vi "IC measurment N6972A - Rohan version - 24.06 WHILELOOP.vi"() -> ()   [LabVIEW 2022 SP3]
doc: "This example demonstrates how to configure a list in current priority mode."
uses:
  <vilib>/Analysis/baseanly.llb/Mean (DBL).vi
  <instrlib>/Agilent 34420/Public/Data/Read (Multiple Points).vi
  <instrlib>/Agilent N6900 N7900 Series/Agilent N6900 N7900 Series.lvlib
  <instrlib>/Agilent 34420/Agilent 34420.lvlib
  <vilib>/Analysis/NI_AALBase.lvlib
  <vilib>/Utility/TDMS File Viewer/NI_TDMS File Viewer.lvlib
panel:
  out "Boolean":bool
  out "String":string="WARNING: FILE PATH EXISTS"
  in  "Path":path=path "C:/Users/kumarr3/OneDrive - Victoria University of Wellington - STAFF/Documents/DataFiles/NoLoad" caption="Load File Path or Directory"
  in  "Conduct Experiment\n\n\nLoad Experiment":bool
  in  "relative path (file or folder)":path=path "Test.tdms"
  in  "base path":path=path "C:/Users/kumarr3/OneDrive - Victoria University of Wellington - STAFF/Documents/DataFiles"
  in  "Tab Control":T1(tab)
  in  "N6972A VISA resource name":refnum<visa-resource-name>="USB0::0x0957::0x3407::MY63000447::INSTR"
  in  "Current Priority Voltage Limit":dbl=1.0
  in  "34420A VISA resource name":refnum<visa-resource-name>="COM3"
  in  "Resolution (1E-9)":dbl=1e-09
  in  "Manual Range (0.001)":dbl=0.001
  in  "Auto Range (T: Enable)":bool=TRUE
  in  "Serial Configuration":T2={"Baud Rate"=9600, "Parity"=0, "Data Bits"=8} {"Data Bits" items=["7"=7, "8"=8]; "Parity" items=["None", "Odd", "Even", "Mark", "Space"]; "Baud Rate" items=["300"=300, "600"=600, "1200"=1200, "2400"=2400, "4800"=4800, "9600"=9600]}
  in  "Function (0: DC Volts)":u16(ring) items=["DC Volts", "DC Voltage Ratio", "DC Voltage Difference", "2 Wire Resistance", "4 Wire Resistance", "Temperature"]
  in  "Channel (1: Channel 1)":u16(ring)=1 items=["Channel 1"=1, "Channel 2"=2]
  in  "Filter On/Off":string(combo)="OFF"
  in  "Voltmeter Offset Sample Count":i32=10
  in  "Integration Time (4: 10 NPLCs)":u16(ring)=4 items=["0.02 NPLC", "0.2 NPLC", "1 NPLC", "2 NPLCs", "10 NPLCs", "20 NPLCs", "100 NPLCs", "200 NPLCs"]
  out "CURRENT RUN":string
  out "Waveform Chart":dbl(graph)
  in  "Measure Temperature?":bool
  out "Temperature Chart":dbl[](graph)=[25.735546538805686]
  out "?":string
  out "Progress Bar":dbl(slide) scale=0.0..1000.0
  in  "Minutes  / Seconds":bool
  in  "Hours / Minutes":bool
  in  "RUN MULTIPLE MEASUREMENTS":bool
  in  "Measurement Interval":dbl
  in  "Total Measurement Time":dbl
  out "XY Graph":cluster{dbl[], dbl[]}(graph)
  out "RMS Current":dbl
  out "uV/cm":dbl
  out "Voltmeter offset (µV)":dbl format="%e"
  out "Current array":dbl[](array[numeric])
  out "Voltage  array":dbl[](array[numeric])
  out "?":bool
  in  "Volt. Tap threshold (uV/cm)":dbl=0.25 format="%.2f"
  in  "Current increment above µV threshold [A]":dbl=0.1 format="%.2f"
  out "?":bool
  in  "Current increment 2 [A]":dbl=0.2 format="%.2f"
  in  "Current limit 1 [A]":dbl=38.0 format="%.2f"
  in  "Initial Current increment  [A]":dbl=5.0 format="%.2f"
  out "Max volt. reached":bool
  out "Max. current reached":bool
  in  "Max. Volt. Tap Voltage (uV/cm)":dbl=10.0
  in  "Maximum current (A)":dbl=48.0
  in  "Volt. Tap Distance (cm)":dbl=1.6
  in  "stop":bool
  out "Calibrating Offset?":bool
  out "Offset V vals":dbl[](array[numeric])
  out "Terminated Temp Msre":bool=TRUE
  in  "Temperature Reading Iterval(s)":u32=1
  in  "Ramp interval (s)":u32
  out "Start Time":timestamp
  out "Experiment Elapsed Time":string
  out "Experiment Remaining Time":string
  out "Waiting time elapsed":string
  in  "Number of Repeats":i32=1
  out "n Values":cluster{timestamp[], dbl[]}(graph)
  out "Ic Values":cluster{timestamp[], dbl[]}(graph)
  out "Fitting Status":string
  out "median Ic":dbl format="%0.2f"
  out "Current Run":cluster{dbl[], dbl[]}(graph) caption="XY Graph"
  out "Historial Results":cluster{dbl[], dbl[]}[](graph) caption="XY Graph"
  out "Ic Array":dbl[](array[numeric])
  out "n Array":dbl[](array[numeric])
  out "mean Ic":dbl format="%0.2f"
  out "mean n":dbl format="%0.2f"
  out "median n":dbl format="%0.2f"
  out "XY Graph 2":cluster{timestamp[], dbl[]}(graph)
  out "median n":dbl format="%0.2f"
  out "n Values Graph":cluster{timestamp[], dbl[]}(graph)
  out "Ic Values Graph":cluster{timestamp[], dbl[]}(graph)
  out "n Array":dbl[](array[numeric])
  out "Ic Array":dbl[](array[numeric])
  out "mean n":dbl format="%0.2f"
  out "mean Ic (A)":dbl format="%0.2f"
  out "Historical Data":cluster{"Array":dbl[], "Array":dbl[]}[](graph)
  out "Number of Runs":dbl
  out "Experiment Description":variant
  out "median Ic (A)":dbl format="%0.2f"
  out "current time":timestamp
  # "Ic Test Controls"
  # "Experiment Control"
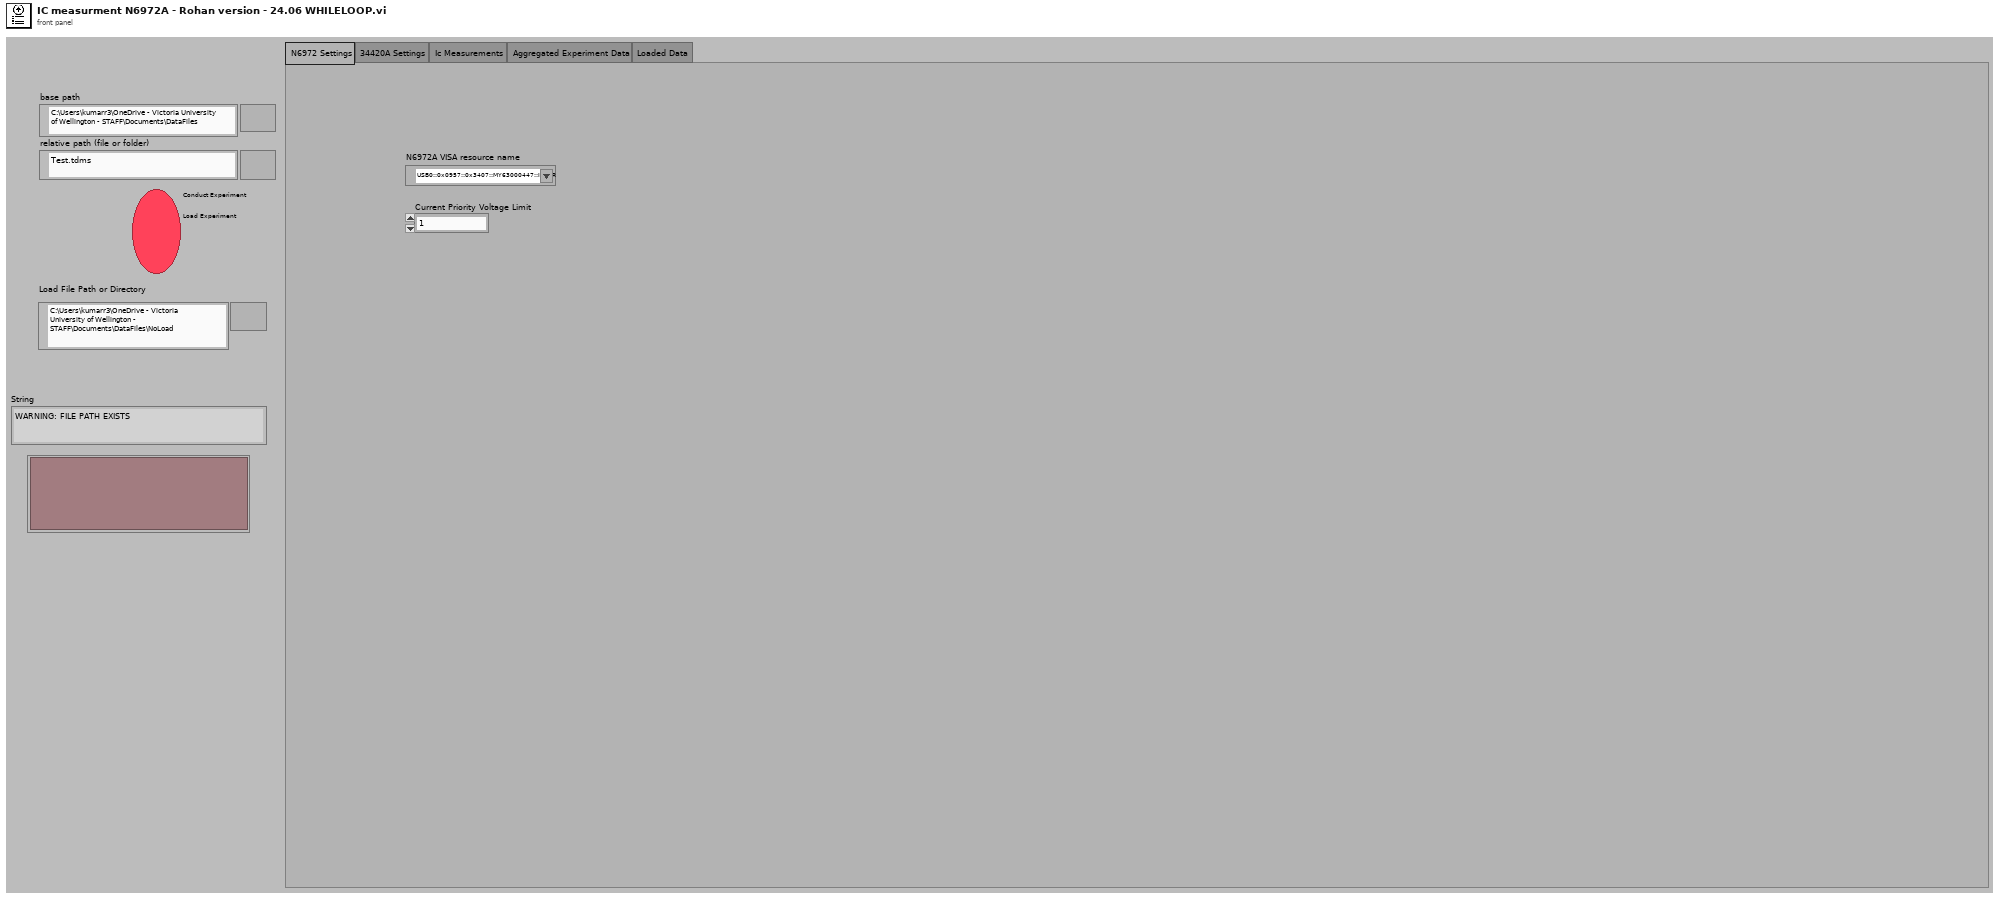
[diagram p1: front panel]
types:
  T1 = enum32{"N6972 Settings", "34420A Settings", "Ic Measurements", "Aggregated Experiment Data", "Loaded Data"}
  T2 = cluster{"Baud Rate":u32, "Parity":u16, "Data Bits":u16}
  T3 = enum16{"open", "open or create", "create or replace", "create", "open (read-only)"}
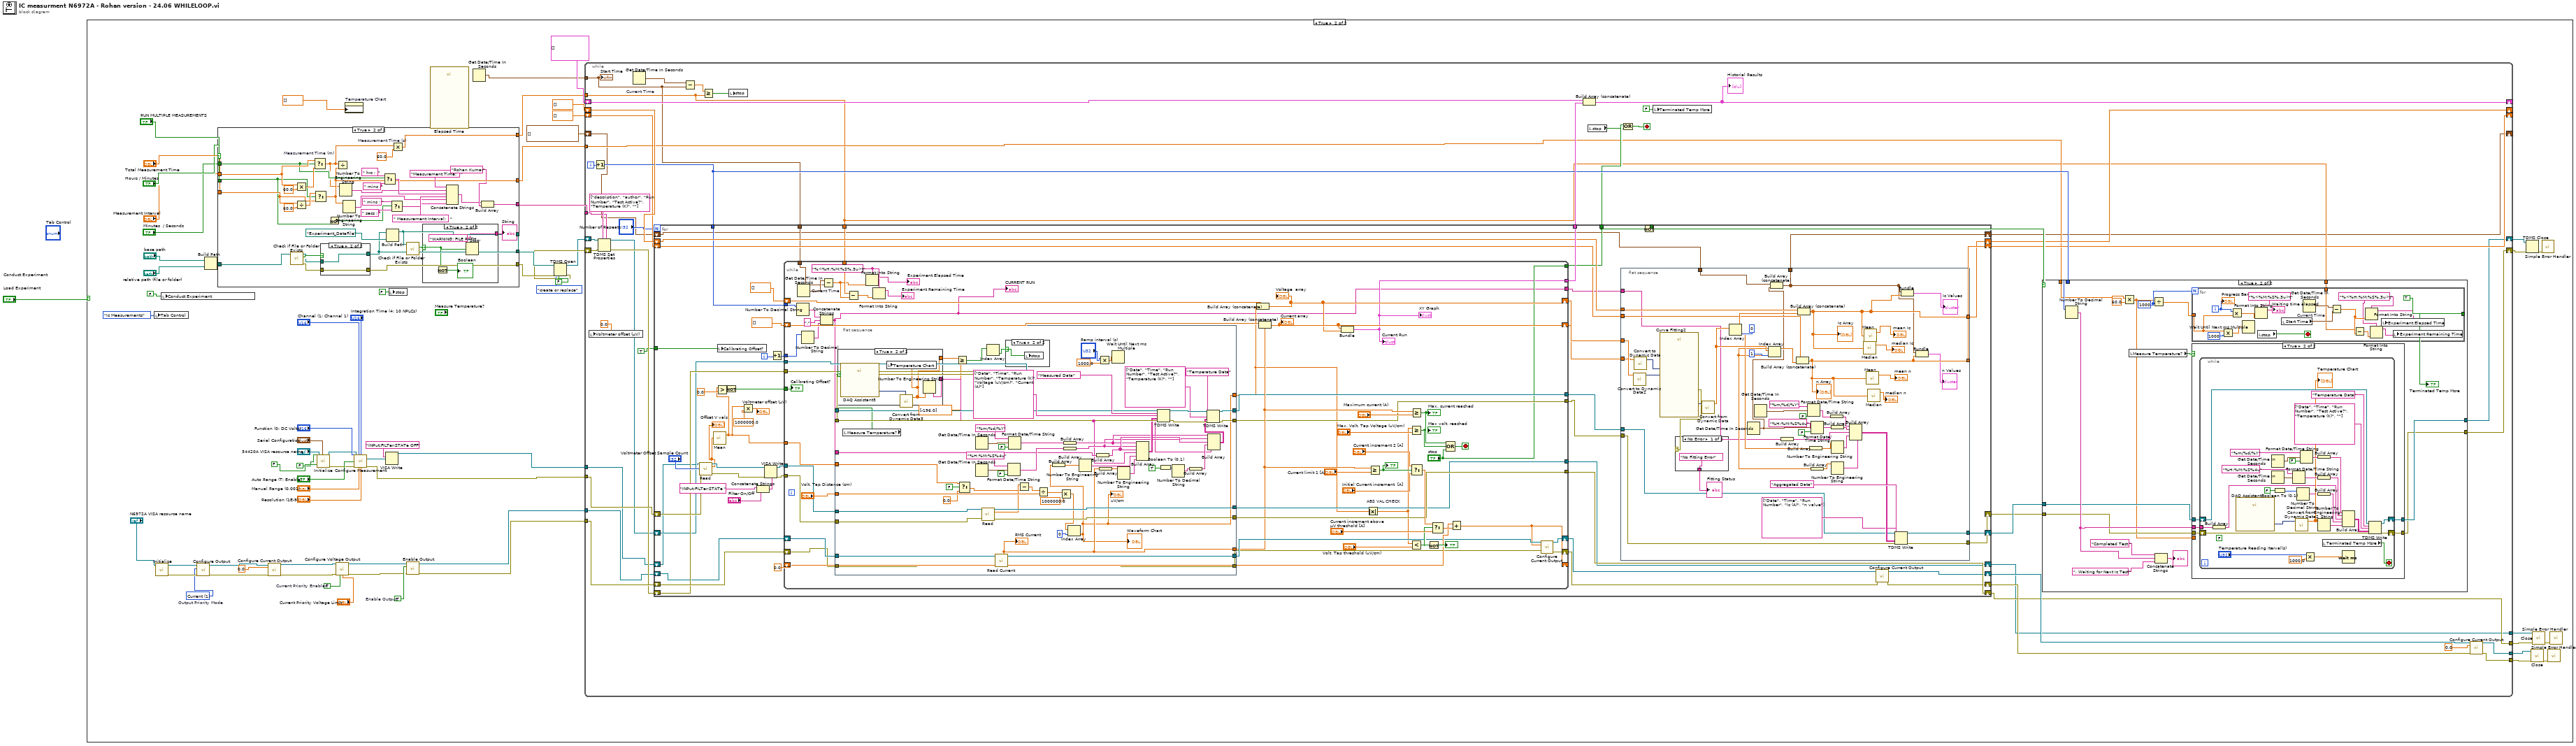
[diagram p0: block diagram]
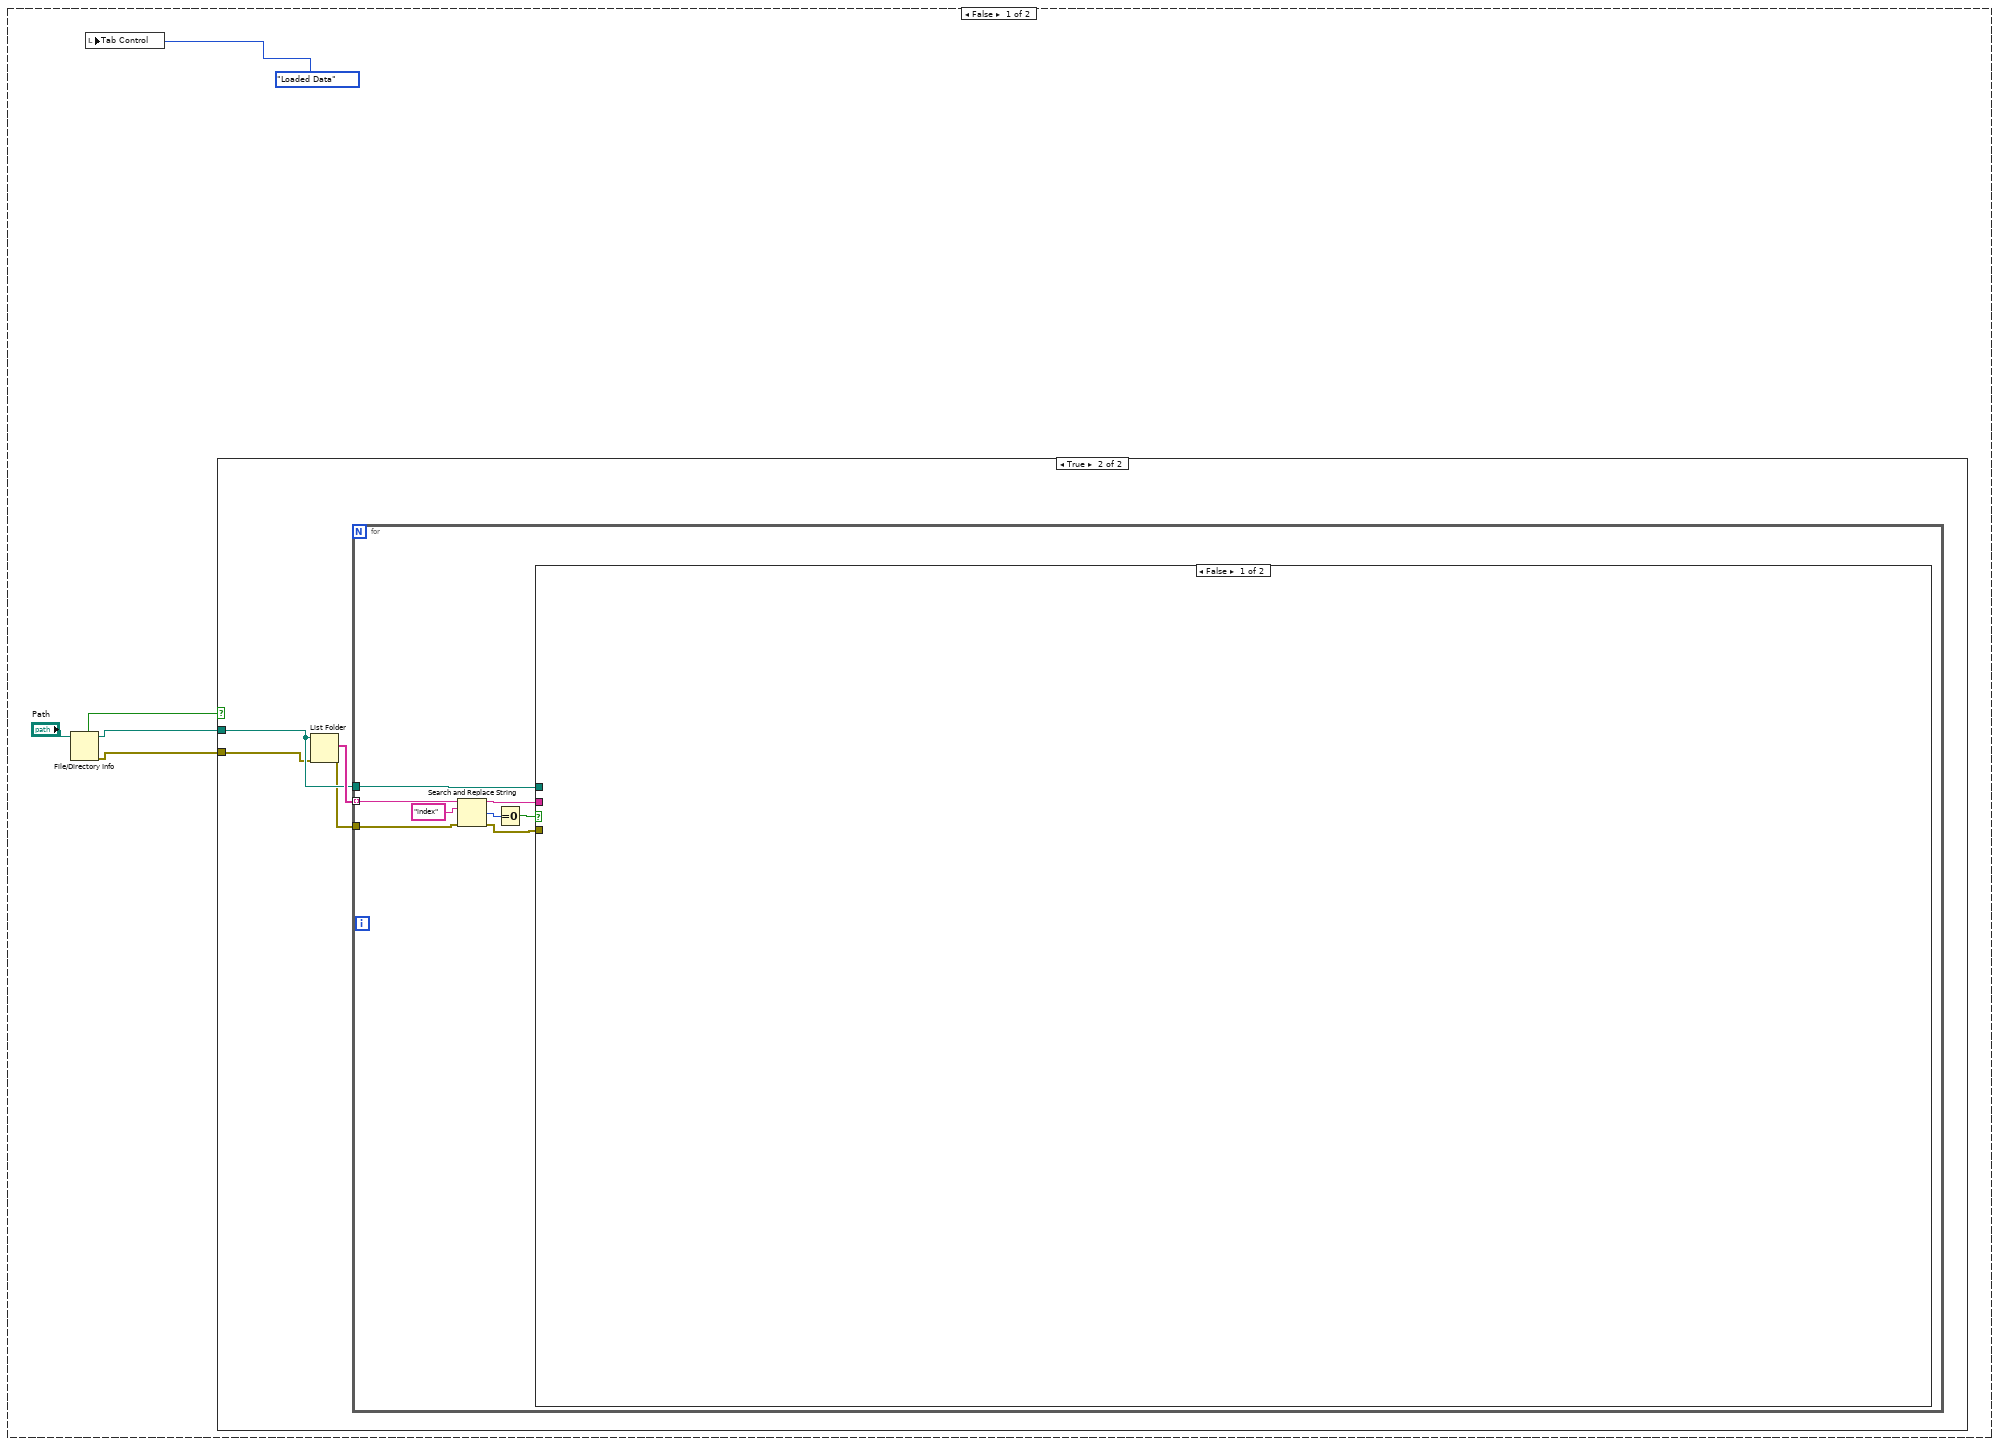
[diagram p2: hidden frame]
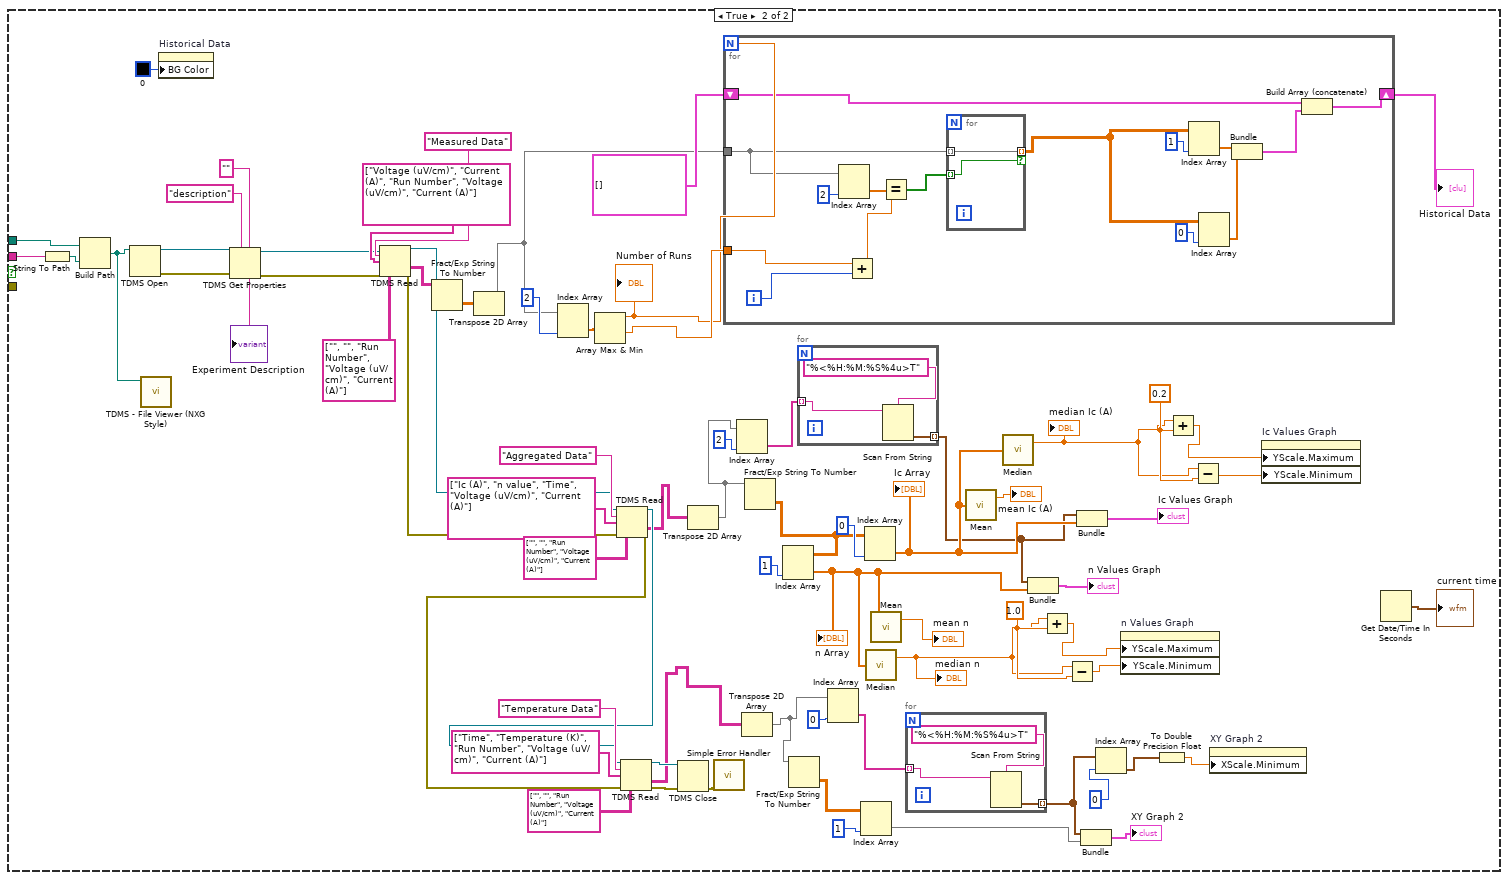
[diagram p4: hidden frame]
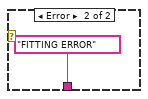
[diagram p5: hidden frame]
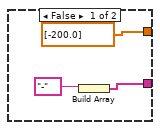
[diagram p7: hidden frame]
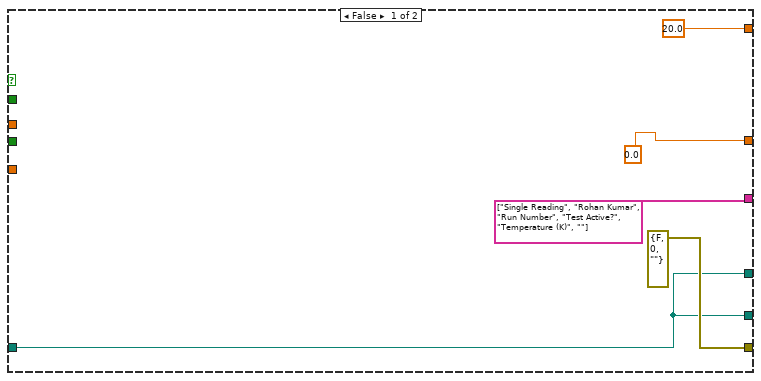
[diagram p10: hidden frame]
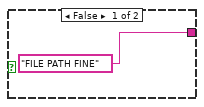
[diagram p11: hidden frame]
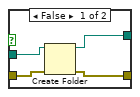
[diagram p12: hidden frame]
diagram:
  n1 = case shown="True" "Conduct Experiment\n\n\nLoad Experiment" {
    frame False {
      n2 = File/Directory Info(path="Path") -> (path out=w5:path, directory=w4:bool, error out=w3:errorcluster)  [unwired: 1 in, 4 out]
      n3 = local write "Tab Control"(T1."Loaded Data" ("Tab Control")) -> ()
      n4 = case shown="True" w4 {
        tunnel: w5 -> [_ w9]
        tunnel: w3 -> [_ w8]
        frame False {
        }
        frame True {
          n5 = List Folder(path=w9, error in=w8) -> (filenames=w10:string[], error out=w7:errorcluster)  [unwired: 2 in, 2 out]
          n6 = for {
            tunnel: w10 -> [w18] mode=indexing
            tunnel: w9 -> [w14]
            tunnel: w7 -> [w12]
            n7 = Search and Replace String(input string=w18, search string="index", error in=w12) -> (result string=w13:string, number of replacements=w16:i32, error out=w11:errorcluster)  [unwired: 5 in, 1 out]
            n8 = Equal To 0?(x=w16) -> (x = 0?=w15:bool)
            n9 = case shown="False" w15 {
              tunnel: w13 -> [_ w90]
              tunnel: w14 -> [_ w89]
              tunnel: w11 -> [_ _]
              frame False {
              }
              frame True {
                w27 = 1.0
                w29 = 0.2
                n10 = String To Path(string=w90) -> (path=w88:path)
                n11 = Build Path(base path=w89, name or relative path=w88) -> (appended path=w19:path)
                n12 = TDMS Open(11:w19) -> (0:w66:errorcluster, 3:w67:refnum<k34>)  [unwired: 6 in]
                n13 = call <vilib>:"TDMS - File Viewer (NXG Style).vi"("file in"=w19) -> ()  [unwired: 9 in, 2 out]
                n14 = property on="Historical Data" class="XYGraph (strict)"("BG Color"=u32 0 ("Plot Area:Colors:BG Color")) -> ()  [unwired: 2 in, 2 out]
                n15 = TDMS Get Properties(5:"", 7:"description", 8:w66, 11:w67) -> (0:w64:errorcluster, 3:w65:refnum<k34>, 4:→"Experiment Description":string)  [unwired: 2 in, 3 out]
                n16 = TDMS Read(0:w65, 5:"Measured Data" ("group name in"), 7:string[] ["Voltage (uV/cm)", "Current (A)", "Run Number", "Voltage (uV/cm)", "Current (A)"] ("channel name(s) in (Untitled)"), 11:w64, 12:string[][] [["", "", "Run Number", "Voltage (uV/cm)", "Current (A)"]] ("channel name(s) in (Untitled)")) -> (4:w54:refnum<k34>, 10:w84:string[][], 15:w53:errorcluster)  [unwired: 3 in, 3 out]
                n17 = Fract/Exp String To Number(string=w84) -> (number=w83:dbl[][])  [unwired: 3 in, 1 out]
                n18 = Transpose 2D Array(2D array=w83) -> (transposed array=w69:dbl[][])
                n19 = Index Array(array=w69, index (col)=2 ("disabled index (col)")) -> (element=w74:dbl[])  [unwired: 1 in]
                n20 = Array Max & Min(array=w74) -> (max value=w72:dbl, min value=w73:dbl)  [unwired: 2 out]
                "Number of Runs" <- w72
                n21 = TDMS Read(0:w54, 5:"Aggregated Data" ("group name in"), 7:string[] ["Ic (A)", "n value", "Time", "Voltage (uV/cm)", "Current (A)"] ("channel name(s) in (Untitled)"), 11:w53, 12:string[][] [["", "", "Run Number", "Voltage (uV/cm)", "Current (A)"]] ("channel name(s) in (Untitled)")) -> (4:w52:refnum<k34>, 10:w34:string[][], 15:w51:errorcluster)  [unwired: 3 in, 3 out]
                n22 = TDMS Read(0:w52, 5:"Temperature Data" ("group name in"), 7:string[] ["Time", "Temperature (K)", "Run Number", "Voltage (uV/cm)", "Current (A)"] ("channel name(s) in (Untitled)"), 11:w51, 12:string[][] [["", "", "Run Number", "Voltage (uV/cm)", "Current (A)"]] ("channel name(s) in (Untitled)")) -> (4:w56:refnum<k34>, 10:w48:string[][], 15:w55:errorcluster)  [unwired: 3 in, 3 out]
                n23 = TDMS Close(8:w55, 11:w56) -> (0:w60:errorcluster)  [unwired: 1 out]
                n24 = Transpose 2D Array(2D array=w34) -> (transposed array=w33:string[][])
                n25 = call <vilib>:"Simple Error Handler.vi"("error in (no error)"=w60) -> ()  [unwired: 2 in, 7 out]
                n26 = for {
                  N: w72 -> [_]
                  tunnel: w69 -> [w105]
                  tunnel: w73 -> [w103]
                  shift-right: [w97] -> w70
                  shift-left: cluster{dbl[], dbl[]}[] [] -> [w99]
                  i -> [w111]
                  n27 = Index Array(array=w105, index (col)=2 ("disabled index (col)")) -> (element=w106:dbl[])  [unwired: 1 in]
                  n28 = Add(x=w103, y=w111) -> (x+y=w104:dbl)
                  n29 = Equal?(x=w106, y=w104) -> (x = y?=w101:bool[])
                  n30 = for {
                    tunnel: w101 -> [w112] mode=indexing
                    tunnel: w105 -> [w113] mode=indexing
                    tunnel: [w113] -> w102 mode=indexing if=w112
                  }
                  n31 = Index Array(array=w102, index (col)=1 ("disabled index (col)")) -> (element=w108:dbl[])  [unwired: 1 in]
                  n32 = Index Array(array=w102, index (col)=0 ("disabled index (col)")) -> (element=w107:dbl[])  [unwired: 1 in]
                  n33 = Bundle(w108, w107) -> (w98:cluster{dbl[], dbl[]})  [unwired: 1 in]
                  n34 = Build Array (concatenate)(w99, w98) -> (w97:cluster{dbl[], dbl[]}[])
                }
                "Historical Data" <- w70
                n35 = Index Array(array=w33, index (col)=2 ("disabled index (col)")) -> (element=w40:string[])  [unwired: 1 in]
                n36 = Transpose 2D Array(2D array=w48) -> (transposed array=w45:string[][])
                n37 = Fract/Exp String To Number(string=w33) -> (number=w32:dbl[][])  [unwired: 3 in, 1 out]
                n38 = Index Array(array=w32, index (col)=1 ("disabled index (col)")) -> (element=w39:dbl[])  [unwired: 1 in]
                "n Array" <- w39
                n39 = Fract/Exp String To Number(string=w45) -> (number=w47:dbl[][])  [unwired: 3 in, 1 out]
                n40 = for {
                  tunnel: w40 -> [w93] mode=indexing
                  tunnel: [w91] -> w36 mode=indexing
                  n41 = Scan From String(format string="%<%H:%M:%S%4u>T" ("time format string (%c)"), input string=w93) -> (output 1=w91:timestamp)  [unwired: 3 in, 3 out]
                }
                n42 = Index Array(array=w45, index (col)=0 ("disabled index (col)")) -> (element=w44:string[])  [unwired: 1 in]
                n43 = Index Array(array=w47, index (col)=1 ("disabled index (col)")) -> (element=w43:dbl[])  [unwired: 1 in]
                n44 = Index Array(array=w32, index (col)=0 ("disabled index (col)")) -> (element=w37:dbl[])  [unwired: 1 in]
                "Ic Array" <- w37
                n45 = call <vilib>:"Median.vi"("X"=w39) -> ("median"=w24:dbl)  [unwired: 1 out]
                "median n" <- w24
                n46 = call-poly <vilib>:"Mean.vi"("X"=w39) -> ("mean"=→"mean n":dbl)  [unwired: 1 out]
                n47 = for {
                  tunnel: w44 -> [w96] mode=indexing
                  tunnel: [w94] -> w23 mode=indexing
                  n48 = Scan From String(format string="%<%H:%M:%S%4u>T" ("time format string (%c)"), input string=w96) -> (output 1=w94:timestamp)  [unwired: 3 in, 3 out]
                }
                n49 = call-poly <vilib>:"Mean.vi"("X"=w37) -> ("mean"=→"mean Ic (A)":dbl)  [unwired: 1 out]
                n50 = call <vilib>:"Median.vi"("X"=w37) -> ("median"=w28:dbl)  [unwired: 1 out]
                "median Ic (A)" <- w28
                n51 = Bundle(w36, w39) -> (→"n Values Graph":cluster{timestamp[], dbl[]})  [unwired: 1 in]
                n52 = Add(x=w24, y=w27) -> (x+y=w26:dbl)
                n53 = Subtract(x=w24, y=w27) -> (x-y=w25:dbl)
                n54 = Bundle(w36, w37) -> (→"Ic Values Graph":cluster{timestamp[], dbl[]})  [unwired: 1 in]
                n55 = Bundle(w23, w43) -> (→"XY Graph 2":cluster{timestamp[], dbl[]})  [unwired: 1 in]
                n56 = Index Array(array=w23, index=0 ("disabled index (col)")) -> (element=w21:timestamp)
                n57 = property on="n Values Graph" class="XYGraph (strict)"("YScale.Maximum"=w26, "YScale.Minimum"=w25) -> ()  [unwired: 2 in, 2 out]
                n58 = To Double Precision Float(number=w21) -> (double precision float=w20:dbl)
                n59 = Add(x=w28, y=w29) -> (x+y=w30:dbl)
                n60 = Subtract(x=w28, y=w29) -> (x-y=w31:dbl)
                n61 = property on="XY Graph 2" class="XYGraph (strict)"("XScale.Minimum"=w20) -> ()  [unwired: 2 in, 2 out]
                n62 = property on="Ic Values Graph" class="XYGraph (strict)"("YScale.Maximum"=w30, "YScale.Minimum"=w31) -> ()  [unwired: 2 in, 2 out]
                n63 = Get Date/Time In Seconds() -> (seconds since 1Jan1904=→"current time":timestamp)
              }
            }
          }
        }
      }
    }
    frame True {
      w174 = TRUE  # Enable Output
      w171 = TRUE  # Current Priority Enabled
      w178 = u16 1 items=["Voltage", "Current"]  # Output Priority Mode
      n64 = local write "Tab Control"(T1."Ic Measurements" ("Tab Control")) -> ()
      n65 = call <instrlib>:"Initialize.vi"("VISA resource name"="N6972A VISA resource name") -> ("error out"=w179:errorcluster, "VISA resource name out"=w180:refnum<visa-resource-name>)  [unwired: 9 in]
      n66 = local write "Conduct Experiment\n\n\nLoad Experiment"(FALSE) -> ()
      n67 = call <instrlib>:"Configure Output.vi"("error in (no error)"=w179, "Output Priority Mode (0: Voltage)"=w178, "VISA resource name"=w180) -> ("error out"=w176:errorcluster, "VISA resource name out"=w177:refnum<visa-resource-name>)  [unwired: 7 in]
      n68 = Build Path(base path="base path", name or relative path="relative path (file or folder)") -> (appended path=w133:path)
      n69 = case shown="True" "RUN MULTIPLE MEASUREMENTS" {
        tunnel: "Total Measurement Time" -> [_ w558]
        tunnel: "Measurement Interval" -> [_ w555]
        tunnel: [0.0 ("Measurement Interval (Minutes)") w544] -> w132
        tunnel: w133 -> [w528 w564]
        tunnel: [w528 w538] -> w127
        tunnel: [errorcluster {"status"=FALSE, "code"=0, "source"=""} ("error out") w561] -> w129
        tunnel: "Hours / Minutes" -> [_ w545]
        tunnel: "Minutes  / Seconds" -> [_ w535]
        tunnel: [w528 w554] -> _
        tunnel: [string[] ["Single Reading", "Rohan Kumar", "Run Number", "Test Active?", "Temperature (K)", ""] ("channel name(s) in (Untitled)") w539] -> w120
        tunnel: [20.0 ("Measurement Interval (Minutes)") w532] -> w115
        frame False {
        }
        frame True {
          n70 = call <vilib>:"Check if File or Folder Exists.vi"("path"=w564) -> ("error out"=w562:errorcluster, "file or folder exists?"=w563:bool, "dup path"=w560:path)  [unwired: 8 in]
          n71 = Multiply(x=w558, y=60.0) -> (x*y=w557:dbl)
          n72 = Divide(x=w555, y=60.0) -> (x/y=w556:dbl)
          n73 = Select "Measurement Time (m)"(t=w558, s=w545, f=w557) -> (s? t:f=w531:dbl)
          n74 = Select(t=w556, s=w535, f=w555) -> (s? t:f=w544:dbl)
          n75 = case shown="True" w563 {
            tunnel: w562 -> [w574 w575]
            tunnel: [w573 w575] -> w561
            tunnel: [w572 w576] -> w554
            tunnel: w560 -> [w571 w576]
            frame False {
              n76 = Create Folder(path (use dialog)=w571, error in=w574) -> (created path=w572:path, error out=w573:errorcluster)  [unwired: 1 in, 1 out]
            }
            frame True {
            }
          }
          n77 = Not(x=w535) -> (.not. x?=w534:bool)
          n78 = Divide(x=w531, y=w544) -> ()  [unwired: 1 out]
          n79 = Number To Engineering String(4:w531) -> (0:w542:string)  [unwired: 3 in]
          n80 = Number To Engineering String(4:w544) -> (0:w543:string)  [unwired: 3 in]
          n81 = Select(t=" hrs ;  ", s=w545, f=" mins ;") -> (s? t:f=w548:string)
          n82 = Build Path(base path=w554, name or relative path=path "Experiment_DataFile") -> (appended path=w538:path)
          n83 = Select(t=" mins ; ", s=w534, f=" secs ; ") -> (s? t:f=w546:string)
          n84 = Multiply "Measurement Time (s)"(x=w531, y=60.0) -> (x*y=w532:dbl)
          n85 = call <vilib>:"Check if File or Folder Exists.vi"("path"=w538) -> ("file or folder exists?"=w537:bool)  [unwired: 8 in, 2 out]
          n86 = case shown="True" w537 {
            selector: w537 -> [_ w569]
            tunnel: ["FILE PATH FINE" "WARNING: FILE PATH EXISTS"] -> w536
            frame False {
            }
            frame True {
              n87 = Not(x=w569) -> (.not. x?=→"Boolean":bool)
              n88 = Stop(stop? (T)=w569) -> ()
            }
          }
          "String" <- w536
          n89 = Concatenate Strings("Measurement Time:   ", w542, w548, " Measurement Interval:   ", w543, w546) -> (w540:string)
          n90 = Build Array(w540, "Rohan Kumar") -> (w539:string[])
        }
      }
      n91 = call <instrlib>:"Configure Current Output.vi"("VISA resource name"=w177, "Current Immediate Amplitude (0 A)"=0.0, "error in (no error)"=w176) -> ("VISA resource name out"=w172:refnum<visa-resource-name>, "error out"=w173:errorcluster)  [unwired: 11 in]
      n92 = call <instrlib>:"Initialize.vi"("Serial Configuration"="Serial Configuration", "Reset (True)"=FALSE, "ID Query (True)"=FALSE, "VISA resource name"="34420A VISA resource name") -> ("error out"=w162:errorcluster, "VISA resource name out"=w161:refnum<visa-resource-name>)  [unwired: 6 in]
      n93 = call <instrlib>:"Configure Voltage Output.vi"("VISA resource name"=w172, "error in (no error)"=w173, "Enable Current Priority (False)"=w171, "Current Priority Voltage Limit (25V)"="Current Priority Voltage Limit") -> ("VISA resource name out"=w169:refnum<visa-resource-name>, "error out"=w168:errorcluster)  [unwired: 10 in]
      n94 = property on="Temperature Chart" class="WFChart (strict)"("History Data"=dbl[] []) -> ()  [unwired: 2 in, 2 out]
      n95 = call <instrlib>:"Configure Measurement.vi"("VISA resource name"=w161, "Channel (1: Channel 1)"="Channel (1: Channel 1)", "Integration Time (4: 10 NPLCs)"="Integration Time (4: 10 NPLCs)", "Function (0: DC Volts)"="Function (0: DC Volts)", "Auto Range (T:Enable)"="Auto Range (T: Enable)", "error in (no error)"=w162, "Manual Range (0.001)"="Manual Range (0.001)", "Resolution (1E-9)"="Resolution (1E-9)") -> ("VISA resource name out"=w156:refnum<visa-resource-name>, "error out"=w149:errorcluster)  [unwired: 6 in]
      n96 = VISA Write(VISA resource name=w156, write buffer="INPut:FILTer:STATe OFF") -> (VISA resource name out=w150:refnum<visa-resource-name>)  [unwired: 1 in, 2 out]
      n97 = local write "stop"(FALSE ("stop")) -> ()
      n98 = call <instrlib>:"Enable Output.vi"("error in (no error)"=w168, "Enable Output (F: Disable)"=w174, "VISA resource name"=w169) -> ("error out"=w153:errorcluster, "VISA resource name out"=w154:refnum<visa-resource-name>)  [unwired: 7 in]
      n99 = call "Elapsed Time"() -> ()  [unwired: 12 in, 8 out]
      n100 = Get Date/Time In Seconds() -> (seconds since 1Jan1904=w116:timestamp)
      n101 = TDMS Open(6:FALSE ("disable buffering (T)"), 8:w129, 10:T3."create or replace" ("operation"), 11:w127) -> (0:w126:errorcluster, 3:w125:refnum<k34>)  [unwired: 3 in]
      n102 = while {
        tunnel: w154 -> [w184]
        tunnel: w153 -> [w223]
        tunnel: w132 -> [w192]
        tunnel: w150 -> [w185]
        tunnel: w149 -> [w221]
        tunnel: [w220] -> w147
        tunnel: [w219] -> w146
        tunnel: [w218] -> w144
        tunnel: [w213] -> w143
        shift-right: [w197] -> _
        shift-left: cluster{dbl[], dbl[]}[] [] -> [w215]
        shift-right: [w200] -> _
        shift-left: dbl[] [] -> [w214]
        shift-right: [w201] -> _
        shift-left: dbl[] [] -> [w198]
        shift-right: [w195] -> w124
        shift-left: w125 -> [w207]
        shift-right: [w196] -> w131
        shift-left: w126 -> [w206]
        tunnel: w120 -> [w202]
        tunnel: w116 -> [w188]
        tunnel: w115 -> [w187]
        shift-right: [w182] -> _
        shift-left: timestamp[] [] -> [w183]
        i -> [w217]
        stop <- w209 stop-if-true
        n103 = local write "Voltmeter offset (µV)"(0.0 ("Voltmeter offset (v)")) -> ()
        n104 = Increment(x=w217) -> (x+1=w211:i32)
        n105 = TDMS Set Properties(5:w202, 7:string[] ["description", "author", "Run Number", "Test Active?", "Temperature (K)", ""] ("channel name(s) in (Untitled)"), 8:w206, 11:w207) -> (0:w205:errorcluster, 3:w204:refnum<k34>)  [unwired: 2 in, 2 out]
        n106 = Get Date/Time In Seconds "Current Time"() -> (seconds since 1Jan1904=w191:timestamp)
        n107 = for {
          N: "Number of Repeats" -> [_]
          tunnel: [w263] -> w216
          tunnel: [w258] -> w212
          tunnel: w211 -> [w257]
          tunnel: [w255] -> w210
          tunnel: w188 -> [w241]
          tunnel: w187 -> [w240]
          shift-right: [w236] -> w225
          shift-left: w223 -> [w275]
          shift-right: [w242] -> w193
          shift-left: w221 -> [w267]
          shift-right: [w264] -> w218
          shift-left: w205 -> [w254]
          shift-right: [w243] -> w194
          shift-left: w204 -> [w253]
          shift-right: [w252] -> w201
          shift-left: w198 -> [w246]
          shift-right: [w251] -> w200
          shift-left: w214 -> [w260]
          shift-right: [w238] -> w226
          shift-left: w184 -> [w234]
          shift-right: [w259] -> w213
          shift-left: w185 -> [w235]
          shift-right: [w232] -> w182
          shift-left: w183 -> [w233]
          tunnel: TRUE ("x > y?") -> [w231]
          i -> [w227]
          n108 = call-poly <instrlib>:"Read.vi"("VISA resource name"=w235, "Sample Count (1)"="Voltmeter Offset Sample Count", "error in (no error)"=w267) -> ("VISA resource name out"=w272:refnum<visa-resource-name>, "Measurements"=w250:dbl[], "error out"=w273:errorcluster)  [unwired: 10 in]
          "Offset V vals" <- w250
          n109 = call-poly <vilib>:"Mean.vi"("X"=w250) -> ("mean"=w249:dbl)  [unwired: 1 out]
          n110 = Greater?(x=w249, y=0.0) -> (0:w256:bool)
          n111 = local write "Calibrating Offset?"(w231) -> ()
          n112 = Not(x=w256) -> (.not. x?=w230:bool)
          n113 = Multiply(x=w249, y=1000000.0) -> (x*y=→"Voltmeter offset (µV)":dbl)
          n114 = Concatenate Strings("INPut:FILTer:STATe ", "Filter On/Off") -> (w274:string)
          n115 = VISA Write(VISA resource name=w272, write buffer=w274, error in (no error)=w273) -> (VISA resource name out=w265:refnum<visa-resource-name>, error out=w266:errorcluster)  [unwired: 1 out]
          n116 = Increment(x=w227) -> (x+1=w228:i32)
          n117 = while {
            shift-right: [w371] -> w239
            shift-left: w234 -> [w384]
            shift-right: [w369] -> w237
            shift-left: w275 -> [w364]
            shift-right: [w368] -> _
            shift-left: 0.0 -> [w373]
            shift-right: [w354] -> w261
            shift-left: dbl[] [] -> [w367]
            tunnel: [w366] -> w264
            tunnel: [w365] -> w259
            shift-right: [w353] -> w262
            shift-left: dbl[] [] -> [w363]
            tunnel: w265 -> [w357]
            tunnel: w266 -> [w356]
            tunnel: w249 -> [w355]
            tunnel: [w352] -> w245
            tunnel: [w351] -> w244
            tunnel: ["stop"] -> w255
            tunnel: [w345] -> w263
            tunnel: w257 -> [w348]
            tunnel: w254 -> [w347]
            tunnel: w253 -> [w346]
            tunnel: w241 -> [w340]
            tunnel: w240 -> [w338]
            tunnel: w230 -> [w333]
            tunnel: [w329] -> w229
            tunnel: w228 -> [w328]
            stop <- w350 stop-if-true
            w336 = "%<%H:%M:%S%.3u>t" ("format string")
            n118 = Number To Decimal String(number=w348) -> (decimal integer string=w330:string)  [unwired: 1 in]
            n119 = Get Date/Time In Seconds "Current Time"() -> (seconds since 1Jan1904=w341:timestamp)
            n120 = Number To Decimal String(number=w328) -> (decimal integer string=w331:string)  [unwired: 1 in]
            n121 = Concatenate Strings(w330, "." ("string"), w331) -> (w329:string)
            "CURRENT RUN" <- w329
            n122 = Subtract(x=w341, y=w340) -> (x-y=w337:dbl)
            n123 = flat-sequence {
              tunnel: w384 -> [w446]
              tunnel: w364 -> [w445]
              tunnel: [w444] -> w372
              tunnel: [w443] -> w370
              tunnel: [w419] -> w359
              tunnel: [w442] -> w366
              tunnel: [w441] -> w365
              tunnel: [w396] -> w344
              tunnel: "Volt. Tap Distance (cm)" -> [w440]
              tunnel: w357 -> [w436]
              tunnel: w356 -> [w435]
              tunnel: w355 -> [w390]
              tunnel: w346 -> [w432]
              tunnel: [w413] -> w352
              tunnel: w347 -> [w431]
              tunnel: [w410] -> w351
              tunnel: w329 -> [w418]
              frame #0 {
                n124 = local read "Measure Temperature?"() -> (w398:bool)
                n125 = case shown="True" w398 {
                  tunnel: [w449 w453] -> w399
                  tunnel: [dbl[] [-200.0] ("Array") w452] -> w395
                  frame False {
                    n126 = Build Array("-" ("group name")) -> (w449:string[])
                  }
                  frame True {
                    n127 = call "DAQ Assistant3"() -> ("data"=w451:dynamicdata)  [unwired: 17 in, 2 out]
                    n128 = call "Convert from Dynamic Data3"("Dynamic Data Type"=w451) -> ("Array"=w452:dbl[])  [unwired: 3 in]
                    n129 = local write "Temperature Chart"(w452) -> ()
                    n130 = Number To Engineering String(4:w452) -> (0:w453:string[])  [unwired: 3 in]
                  }
                }
                n131 = Greater Or Equal?(x=w395, y=dbl[] [-196.0]) -> (x >= y?=w392:bool[])
                n132 = Select(t=w390, s=FALSE, f=0.0) -> (s? t:f=w389:dbl)
                n133 = Get Date/Time In Seconds() -> (seconds since 1Jan1904=w425:timestamp)
                n134 = Get Date/Time In Seconds() -> (seconds since 1Jan1904=w428:timestamp)
                n135 = call-poly <instrlib>:"Read.vi"("VISA resource name"=w436, "error in (no error)"=w435) -> ("VISA resource name out"=w441:refnum<visa-resource-name>, "Measurements"=w397:dbl[], "error out"=w442:errorcluster)  [unwired: 11 in]
                n136 = Index Array(array=w392) -> (element=w393:bool)  [unwired: 1 in]
                n137 = call <instrlib>:"Read Current.vi"("VISA resource name"=w446, "error in (no error)"=w445) -> ("RMS Current"=w419:dbl, "VISA resource name out"=w444:refnum<visa-resource-name>, "error out"=w443:errorcluster)  [unwired: 6 in, 5 out]
                "RMS Current" <- w419
                n138 = case shown="True" w393 {
                  selector: w393 -> [_ w447]
                  frame False {
                  }
                  frame True {
                    n139 = local write "stop"(w447) -> ()
                  }
                }
                n140 = Format Date/Time String(time format string (%c)="%H:%M:%S%4u", seconds (now)=w428, UTC format=FALSE) -> (date/time string=w423:string)
                n141 = Format Date/Time String(time format string (%c)="%m/%d/%Y", seconds (now)=w425, UTC format=FALSE) -> (date/time string=w424:string)
                n142 = Subtract(x=w397, y=w389) -> (x-y=w437:dbl[])
                n143 = Divide(x=w437, y=w440) -> (x/y=w439:dbl[])
                n144 = Multiply(x=w439, y=1000000.0) -> (x*y=w416:dbl[])
                n145 = Build Array(w424) -> (w401:string[])
                n146 = Build Array(w423) -> (w400:string[])
                n147 = Index Array(array=w416, index=0) -> (element=w396:dbl)
                "uV/cm" <- w396
                "Waveform Chart" <- w396
                n148 = Build Array(w396) -> (w422:dbl[])
                n149 = Number To Engineering String(4:w422) -> (0:w415:string[])  [unwired: 3 in]
                n150 = Build Array(w418) -> (w402:string[])
                n151 = Multiply(x="Ramp interval (s)", y=1000.0) -> (x*y=w386:dbl)
                n152 = Build Array(w419) -> (w420:dbl[])
                n153 = Wait Until Next ms Multiple(millisecond multiple=w386) -> ()  [unwired: 1 out]
                n154 = Number To Engineering String(4:w420) -> (0:w414:string[])  [unwired: 3 in]
                n155 = Build Array(w401, w400, w402, w399, w415, w414) -> (w421:string[][])
                n156 = TDMS Write(0:w432, 5:"Measured Data" ("group name"), 7:string[] ["Date", "Time", "Run Number", "Temperature (K)", "Voltage (uV/cm)", "Current (A)"] ("channel name(s) in (Untitled)"), 9:w421, 11:w431) -> (4:w412:refnum<k34>, 15:w411:errorcluster)  [unwired: 1 in, 2 out]
                n157 = Boolean To (0,1)(Boolean=TRUE) -> (0, 1=w406:i16)
                n158 = Number To Decimal String(number=w406) -> (decimal integer string=w403:string)  [unwired: 1 in]
                n159 = Build Array(w403) -> (w404:string[])
                n160 = Build Array(w401, w400, w402, w404, w399) -> (w405:string[][])
                n161 = TDMS Write(0:w412, 5:"Temperature Data" ("group name"), 7:string[] ["Date", "Time", "Run Number", "Test Active?", "Temperature (K)", ""] ("channel name(s) in (Untitled)"), 9:w405, 11:w411) -> (4:w413:refnum<k34>, 15:w410:errorcluster)  [unwired: 1 in, 2 out]
              }
            }
            n162 = Subtract(x=w338, y=w337) -> (x-y=w335:dbl)
            n163 = Format Into String(format string=w336, w337) -> (resulting string=→"Experiment Elapsed Time":string)  [unwired: 2 in, 1 out]
            n164 = Format Into String(format string=w336, w335) -> (resulting string=→"Experiment Remaining Time":string)  [unwired: 2 in, 1 out]
            n165 = Build Array (concatenate)(w363, w344) -> (w353:dbl[])
            "Voltage  array" <- w353
            n166 = Build Array (concatenate)(w367, w359) -> (w354:dbl[])
            "Current array" <- w354
            n167 = Bundle(w354, w353) -> (w345:cluster{dbl[], dbl[]})  [unwired: 1 in]
            "XY Graph" <- w345
            "Current Run" <- w345
            n168 = Absolute Value "ABS VAL CHECK"(x=w344) -> (abs(x)=w343:dbl)
            n169 = Greater Or Equal?(x=w359, y="Current limit 1 [A]") -> (x >= y?=w375:bool)
            "?" <- w375
            n170 = Greater Or Equal?(x=w343, y="Max. Volt. Tap Voltage (uV/cm)") -> (x >= y?=w360:bool)
            "Max volt. reached" <- w360
            n171 = Less?(x=w343, y="Volt. Tap threshold (uV/cm)") -> (x < y?=w377:bool)
            n172 = Greater Or Equal?(x=w359, y="Maximum current (A)") -> (x >= y?=w362:bool)
            "Max. current reached" <- w362
            n173 = Select(t="Current increment 2 [A]", s=w375, f="Initial Current increment  [A]") -> (s? t:f=w379:dbl)
            n174 = Not(x=w377) -> (.not. x?=→"?":bool)
            n175 = Select(t=w379, s=w377, f="Current increment above µV threshold [A]") -> (s? t:f=w374:dbl)
            n176 = Compound Arithmetic op=OR(w362, w360, "stop") -> (w350:bool)
            n177 = Add(x=w373, y=w374) -> (x+y=w368:dbl)
            n178 = call <instrlib>:"Configure Current Output.vi"("VISA resource name"=w372, "Current Immediate Amplitude (0 A)"=w368, "error in (no error)"=w370) -> ("VISA resource name out"=w371:refnum<visa-resource-name>, "error out"=w369:errorcluster)  [unwired: 11 in]
            "Calibrating Offset?" <- w333
          }
          n179 = flat-sequence {
            tunnel: w262 -> [w325]
            tunnel: w261 -> [w324]
            tunnel: w260 -> [w322]
            tunnel: [w291] -> w243
            tunnel: [w281] -> w252
            tunnel: [w285] -> w251
            tunnel: w246 -> [w294]
            tunnel: w245 -> [w293]
            tunnel: w244 -> [w292]
            tunnel: [w290] -> w242
            tunnel: w233 -> [w286]
            tunnel: [w282] -> w232
            tunnel: w229 -> [w279]
            frame #0 {
              n180 = call "Convert to Dynamic Data2"("Array"=w325) -> ("Dynamic Data Type"=w297:dynamicdata)  [unwired: 3 in]
              n181 = call "Convert to Dynamic Data"("Array"=w324) -> ("Dynamic Data Type"=w296:dynamicdata)  [unwired: 3 in]
              n182 = call "Curve Fitting2"("Locations"=w296, "Signals"=w297) -> ("error out"=w289:errorcluster, "non-linear coefficients"=w295:dynamicdata)  [unwired: 5 in, 3 out]
              n183 = case shown="No Error" w289 {
                tunnel: ["No Fitting Error" ("group name") "FITTING ERROR" ("group name")] -> w288
                frame No Error {
                }
                frame Error {
                }
              }
              "Fitting Status" <- w288
              n184 = call "Convert from Dynamic Data"("Dynamic Data Type"=w295) -> ("Array"=w321:dbl[])  [unwired: 3 in]
              n185 = Index Array(array=w321, index=0) -> (element=w302:dbl)
              n186 = Get Date/Time In Seconds() -> (seconds since 1Jan1904=w283:timestamp)
              n187 = Get Date/Time In Seconds() -> (seconds since 1Jan1904=w313:timestamp)
              n188 = Index Array(array=w321, index=1) -> (element=w287:dbl)
              n189 = Build Array (concatenate)(w286, w283) -> (w282:timestamp[])
              n190 = Build Array(w279) -> (w301:string[])
              n191 = Build Array (concatenate)(w294, w287) -> (w281:dbl[])
              "n Array" <- w281
              n192 = Build Array (concatenate)(w322, w302) -> (w285:dbl[])
              "Ic Array" <- w285
              n193 = Format Date/Time String(time format string (%c)="%m/%d/%Y", seconds (now)=w313, UTC format=FALSE) -> (date/time string=w312:string)
              n194 = Build Array(w302) -> (w308:dbl[])
              n195 = Format Date/Time String(time format string (%c)="%H:%M:%S%4u", seconds (now)=w283, UTC format=FALSE) -> (date/time string=w311:string)
              n196 = Build Array(w287) -> (w306:dbl[])
              n197 = Build Array(w312) -> (w310:string[])
              n198 = Number To Engineering String(4:w308) -> (0:w304:string[])  [unwired: 3 in]
              n199 = Number To Engineering String(4:w306) -> (0:w305:string[])  [unwired: 3 in]
              n200 = Build Array(w311) -> (w309:string[])
              n201 = Build Array(w310, w309, w301, w304, w305) -> (w307:string[][])
              n202 = call <vilib>:"Median.vi"("X"=w285) -> ("median"=→"median Ic":dbl)  [unwired: 1 out]
              n203 = call-poly <vilib>:"Mean.vi"("X"=w285) -> ("mean"=→"mean Ic":dbl)  [unwired: 1 out]
              n204 = call-poly <vilib>:"Mean.vi"("X"=w281) -> ("mean"=→"mean n":dbl)  [unwired: 1 out]
              n205 = call <vilib>:"Median.vi"("X"=w281) -> ("median"=→"median n":dbl)  [unwired: 1 out]
              n206 = TDMS Write(0:w293, 5:"Aggregated Data" ("group name"), 7:string[] ["Date", "Time", "Run Number", "Ic (A)", "n value"] ("channel name(s) in (Untitled)"), 9:w307, 11:w292) -> (4:w291:refnum<k34>, 15:w290:errorcluster)  [unwired: 1 in, 2 out]
              n207 = Bundle(w282, w285) -> (→"Ic Values":cluster{timestamp[], dbl[]})  [unwired: 1 in]
              n208 = Bundle(w282, w281) -> (→"n Values":cluster{timestamp[], dbl[]})  [unwired: 1 in]
            }
          }
          n209 = Not(x=w255) -> (.not. x?=w258:bool)
          n210 = call <instrlib>:"Configure Current Output.vi"("VISA resource name"=w239, "error in (no error)"=w237) -> ("VISA resource name out"=w238:refnum<visa-resource-name>, "error out"=w236:errorcluster)  [unwired: 12 in]
        }
        n211 = Subtract(x=w191, y=w188) -> (x-y=w190:dbl)
        n212 = Greater Or Equal?(x=w190, y=w187) -> (x >= y?=w189:bool)
        n213 = local write "stop"(w189) -> ()
        n214 = Build Array (concatenate)(w215, w216) -> (w197:cluster{dbl[], dbl[]}[])
        "Historial Results" <- w197
        n215 = local read "stop"() -> (w208:bool)
        n216 = Compound Arithmetic op=OR(w210, w208) -> (w209:bool)
        n217 = local write "Terminated Temp Msre"(FALSE ("Terminated Temp Msre")) -> ()
        n218 = case shown="True" w212 {
          tunnel: w211 -> [_ w471]
          tunnel: w194 -> [w455 w465]
          tunnel: w193 -> [w454 w464]
          tunnel: [w455 w463] -> w195
          tunnel: [w454 w462] -> w196
          tunnel: w192 -> [_ w461]
          tunnel: w187 -> [_ w456]
          frame False {
          }
          frame True {
            w469 = 1000
            n219 = Number To Decimal String(number=w471) -> (decimal integer string=w466:string)  [unwired: 1 in]
            n220 = Multiply(x=w461, y=60.0) -> (x*y=w460:dbl)
            n221 = local read "Measure Temperature?"() -> (w459:bool)
            n222 = Divide(x=w460, y=w469) -> (x/y=w468:dbl)
            n223 = Concatenate Strings("Completed Test ", w466, ". Waiting for Next Ic Test" ("Title")) -> (→"?":string)
            n224 = for {
              N: w469 -> [_]
              tunnel: w468 -> [w522]
              tunnel: [TRUE] -> w458
              tunnel: w456 -> [w514]
              i -> [w523]
              stop <- w521 stop-if-true
              w512 = "%<%H:%M:%S%.3u>t" ("format string")
              n225 = Multiply(x=w522, y=u32 1000 ("millisecond multiple")) -> (x*y=w524:dbl)
              n226 = Multiply(x=w523, y=w522) -> (x*y=w511:dbl)
              n227 = Wait Until Next ms Multiple(millisecond multiple=w524) -> ()  [unwired: 1 out]
              n228 = Format Into String(format string="%<%M:%S%.3u>t", w511) -> (resulting string=→"Waiting time elapsed":string)  [unwired: 2 in, 1 out]
              n229 = local read "stop"() -> (w521:bool)
              n230 = local read "Start Time"() -> (w518:timestamp)
              n231 = Get Date/Time In Seconds "Current Time"() -> (seconds since 1Jan1904=w519:timestamp)
              n232 = Subtract(x=w519, y=w518) -> (x-y=w516:dbl)
              n233 = Subtract(x=w514, y=w516) -> (x-y=w515:dbl)
              n234 = Format Into String(format string=w512, w516) -> (resulting string=w517:string)  [unwired: 2 in, 1 out]
              n235 = Format Into String(format string=w512, w515) -> (resulting string=w513:string)  [unwired: 2 in, 1 out]
              n236 = local write "Experiment Elapsed Time"(w517) -> ()
              n237 = local write "Experiment Remaining Time"(w513) -> ()
              "Progress Bar" <- w523
            }
            "Terminated Temp Msre" <- w458
            n238 = case shown="True" w459 {
              tunnel: w466 -> [_ w479]
              tunnel: w465 -> [w474 w478]
              tunnel: w464 -> [w473 w475]
              tunnel: [w474 w477] -> w463
              tunnel: [w473 w476] -> w462
              tunnel: w460 -> [_ _]
              frame False {
              }
              frame True {
                n239 = while {
                  tunnel: w479 -> [w496]
                  shift-right: [w493] -> w477
                  shift-left: w478 -> [w495]
                  shift-right: [w492] -> w476
                  shift-left: w475 -> [w494]
                  stop <- w481 stop-if-true
                  (unwired) FALSE ("UTC format")
                  n240 = Build Array(w496) -> (w484:string[])
                  n241 = call "DAQ Assistant"() -> ("data"=w480:dynamicdata)  [unwired: 17 in, 2 out]
                  n242 = Get Date/Time In Seconds() -> (seconds since 1Jan1904=w502:timestamp)
                  n243 = Get Date/Time In Seconds() -> (seconds since 1Jan1904=w505:timestamp)
                  n244 = Boolean To (0,1)(Boolean=FALSE) -> (0, 1=w485:i16)
                  n245 = Format Date/Time String(time format string (%c)="%H:%M:%S%4u", seconds (now)=w505) -> (date/time string=w500:string)  [unwired: 1 in]
                  n246 = call "Convert from Dynamic Data2"("Dynamic Data Type"=w480) -> ("Array"=w488:dbl[])  [unwired: 3 in]
                  "Temperature Chart" <- w488
                  n247 = Number To Decimal String(number=w485) -> (decimal integer string=w483:string)  [unwired: 1 in]
                  n248 = Format Date/Time String(time format string (%c)="%m/%d/%Y", seconds (now)=w502, UTC format=FALSE) -> (date/time string=w501:string)
                  n249 = Multiply(x="Temperature Reading Iterval(s)", y=1000.0) -> (x*y=w489:dbl)
                  n250 = Build Array(w501) -> (w499:string[])
                  n251 = Build Array(w500) -> (w498:string[])
                  n252 = Build Array(w483) -> (w482:string[])
                  n253 = Number To Engineering String(4:w488) -> (0:w487:string[])  [unwired: 3 in]
                  n254 = local read "Terminated Temp Msre"() -> (w481:bool)
                  n255 = Build Array(w499, w498, w484, w482, w487) -> (w497:string[][])
                  n256 = Wait (ms)(milliseconds to wait=w489) -> ()  [unwired: 1 out]
                  n257 = TDMS Write(0:w495, 5:"Temperature Data" ("group name"), 7:string[] ["Date", "Time", "Run Number", "Test Active?", "Temperature (K)", ""] ("channel name(s) in (Untitled)"), 9:w497, 11:w494) -> (4:w493:refnum<k34>, 15:w492:errorcluster)  [unwired: 1 in, 2 out]
                }
              }
            }
          }
        }
        n258 = call <instrlib>:"Configure Current Output.vi"("VISA resource name"=w226, "Current Immediate Amplitude (0 A)"=0.0, "error in (no error)"=w225) -> ("VISA resource name out"=w219:refnum<visa-resource-name>, "error out"=w220:errorcluster)  [unwired: 11 in]
        "Start Time" <- w188
      }
      n259 = TDMS Close(8:w131, 11:w124) -> (0:w139:errorcluster)  [unwired: 1 out]
      n260 = call <instrlib>:"Close.vi"("error in (no error)"=w147, "VISA resource name"=w146) -> ("error out"=w148:errorcluster)  [unwired: 9 in]
      n261 = call <instrlib>:"Close.vi"("error in (no error)"=w144, "VISA resource name"=w143) -> ("error out"=w145:errorcluster)  [unwired: 9 in]
      n262 = call <vilib>:"Simple Error Handler.vi"("error in (no error)"=w139) -> ()  [unwired: 2 in, 7 out]
      n263 = call <vilib>:"Simple Error Handler.vi"("error in (no error)"=w148) -> ()  [unwired: 4 in, 5 out]
      n264 = call <vilib>:"Simple Error Handler.vi"("error in (no error)"=w145) -> ()  [unwired: 4 in, 5 out]
    }
  }
